vi "Remove Empty Array Elements Return Warning.vi"(8 "error in (no error)":errorcluster, 10 "String Array In":string[](array[string])) -> (0 "error out":errorcluster, 2 "String Array Out":string[](array[string]))   [LabVIEW 2015, in "Case Manipulation.lvlib"]
uses:
  Case Manipulation.lvlib
  <vilib>/ErrorRing/Error Ring.xnode
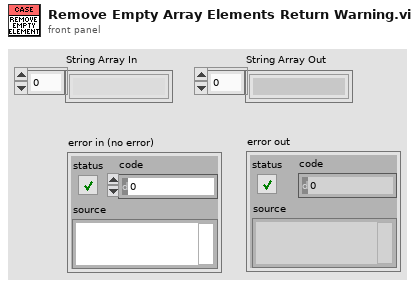
[diagram p1: front panel]
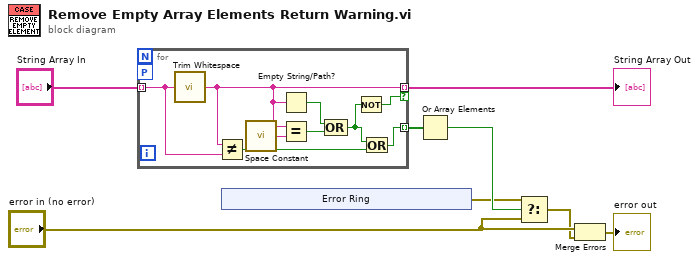
[diagram p0: block diagram]
diagram:
  n1 = for {
    tunnel: "String Array In" -> [w12] mode=indexing
    tunnel: [w13] -> w8 mode=indexing if=w17
    workers-P: _ -> [_]
    tunnel: [w9] -> w7 mode=indexing
    n2 = call <vilib>:"Trim Whitespace.vi"("string"=w12) -> ("trimmed string"=w13:string)  [unwired: 1 in]
    n3 = Not Equal?(x=w13, y=w12) -> (x != y?=w10:bool)
    n4 = call <vilib>:"Space Constant.vi"() -> ("String"=w14:string)
    n5 = Empty String/Path?(string/path=w13) -> (empty?=w16:bool)
    n6 = Equal?(x=w13, y=w14) -> (x = y?=w15:bool)
    n7 = Compound Arithmetic op=OR(w16, w15) -> (w11:bool)
    n8 = Not(x=w11) -> (.not. x?=w17:bool)
    n9 = Or(x=w11, y=w10) -> (x .or. y?=w9:bool)
  }
  "String Array Out" <- w8
  n10 = xnode "Error Ring"() -> ("error out"=w5:errorcluster)
  n11 = Or Array Elements(Boolean array=w7) -> (logical OR=w6:bool)
  n12 = Select(t=w5, s=w6, f="error in (no error)") -> (s? t:f=w2:errorcluster)
  n13 = Merge Errors("error in (no error)", w2) -> (→"error out":errorcluster)
